vi "Array to Spectra (N Ch).vi"(8 "channel names":string[](array[string]), 9 "df":dbl, 10 "f0":dbl, 11 "data":dbl[](array[numeric])) -> (3 "spectra":cluster{"f0":dbl, "df":dbl, "data":dbl[]}[](array[cluster]))   [LabVIEW 2023]
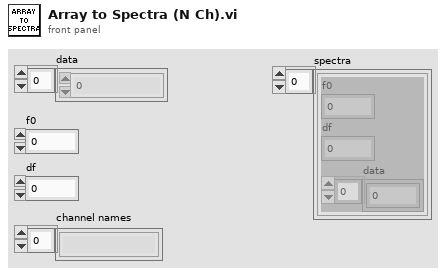
[diagram p1: front panel]
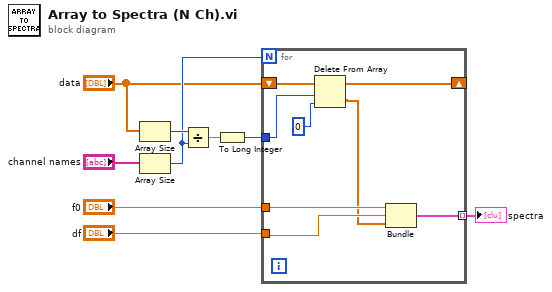
[diagram p0: block diagram]
diagram:
  n1 = Array Size(array="data") -> (size(s)=w9:i32)
  n2 = Array Size(array="channel names") -> (size(s)=w8:i32)
  n3 = Divide(x=w9, y=w8) -> (x/y=w6:dbl)
  n4 = To Long Integer(number=w6) -> (32bit integer=w5:i32)
  n5 = for {
    N: w8 -> [_]
    shift-right: [w12] -> _
    shift-left: "data" -> [w17]
    tunnel: w5 -> [w15]
    tunnel: "f0" -> [w14]
    tunnel: "df" -> [w13]
    tunnel: [w11] -> w1 mode=indexing
    n6 = Delete From Array(array=w17, length=w15, index=0) -> (deleted portion=w10:dbl[], array with subset deleted=w12:dbl[])
    n7 = Bundle("f0"=w14, "df"=w13, "data"=w10) -> (w11:cluster{"f0":dbl, "df":dbl, "data":dbl[]})  [unwired: 1 in]
  }
  "spectra" <- w1
